vi "Async.vi"() -> ()   [LabVIEW 2018]
panel:
  out "Fibonacci(n)":u32
  in  "n":u32
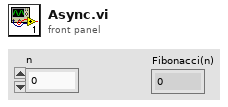
[diagram p1: front panel]
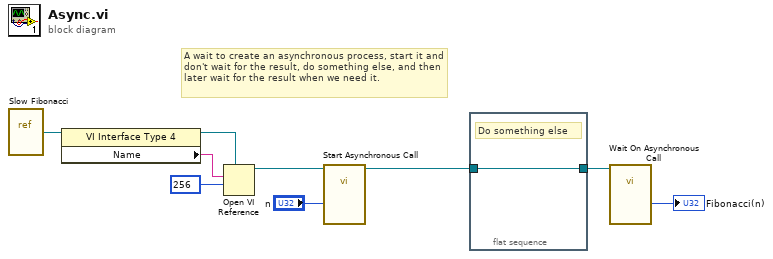
[diagram p0: block diagram]
diagram:
  # "A wait to create an asynchronous process, start it and don't wait for the result, do something else, and then later wait for the result when we need it."
  n1 = vi-ref "Slow Fibonacci.vi"() -> (w4:refnum<vi>)
  n2 = property class="VI Interface Type 4"(reference=w4) -> (reference out=w5:refnum<vi>, "Name"=w6:string)  [unwired: 1 in, 1 out]
  n3 = Open VI Reference(type specifier VI Refnum (for type only)=w5, vi path=w6, options=256) -> (vi reference=w3:refnum<vi>)  [unwired: 3 in, 1 out]
  n4 = call-by-ref "Start Asynchronous Call"(reference=w3, "n"="n") -> (reference out=w2:refnum<vi>)  [unwired: 1 in, 2 out]
  n5 = flat-sequence {
    tunnel: w2 -> [w10]
    tunnel: [w10] -> w1
    frame #0 {
      # "Do something else"
    }
  }
  n6 = call-by-ref "Wait On Asynchronous Call"(reference=w1) -> ("Fibonacci(n)"=→"Fibonacci(n)":u32)  [unwired: 2 in, 2 out]
